vi "多参10分钟延时启动.vi"(11 "启动采配水？":bool) -> ()   [LabVIEW 2016]
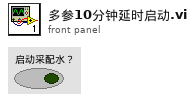
[diagram p1: front panel]
types:
  T1 = cluster{"命令":string, cluster{"starting address":u16, "holding register value":u16}}
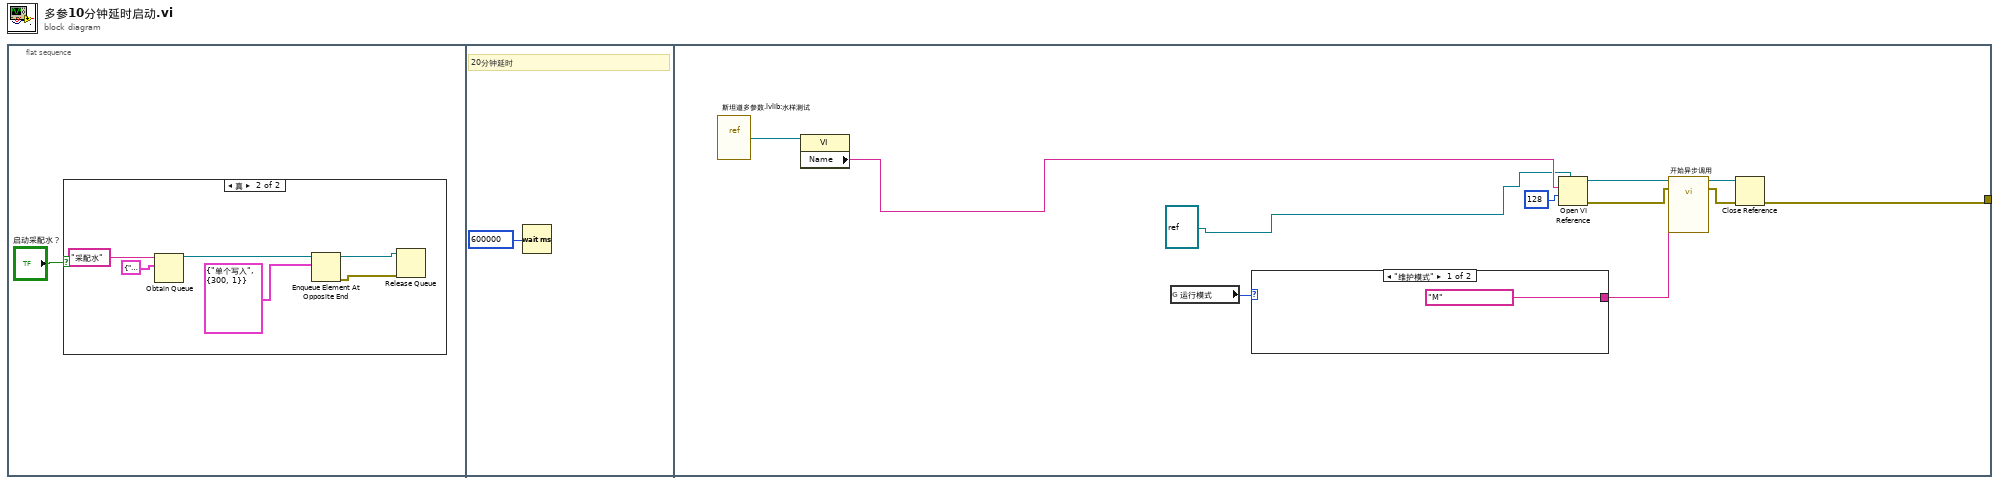
[diagram p0: block diagram]
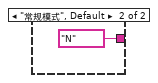
[diagram p3: hidden frame]
diagram:
  n1 = flat-sequence {
    tunnel: [w10] -> _
    frame #0 {
      n2 = case shown="真" "启动采配水？" {
        frame False {
        }
        frame True {
          n3 = Obtain Queue(name (unnamed)="采配水" ("名称（未命名）"), element data type=cluster{"命令":string, "数据":variant} {"命令"="", "数据"=variant}) -> (queue out=w4:refnum<queue>)  [unwired: 3 in, 2 out]
          n4 = Enqueue Element At Opposite End(queue=w4, element=T1 {"命令"="单个写入", {"starting address"=300, "holding register value"=1}} ("元素")) -> (queue out=w3:refnum<queue>, error out=w2:errorcluster)  [unwired: 2 in, 1 out]
          n5 = Release Queue(queue=w3, error in (no error)=w2) -> ()  [unwired: 1 in, 3 out]
        }
      }
    }
    frame #1 {
      # "20分钟延时"
      n6 = Wait (ms)(milliseconds to wait=u32 600000 ("等待时间（毫秒）")) -> ()  [unwired: 1 out]
    }
    frame #2 {
      n7 = vi-ref "斯坦道多参数.lvlib:水样测试.vi"() -> (w19:refnum<vi>)
      n8 = property class="VI"(reference=w19) -> ("Name"=w18:string)  [unwired: 1 in, 2 out]
      n9 = global read "系统设置全局变量.vi" "运行模式"() -> (w14:enum16{"维护模式", "常规模式", "应急模式", "质控模式"})
      n10 = case shown="\"维护模式\"" w14 {
        tunnel: ["M" ("数据标记表") "N" ("数据标记表")] -> w13
        frame "维护模式" {
        }
        frame "常规模式", Default {
        }
      }
      n11 = Open VI Reference(type specifier VI Refnum (for type only)=refnum<vi> refnum, vi path=w18, options=128 ("选项")) -> (vi reference=w16:refnum<vi>, error out=w9:errorcluster)  [unwired: 3 in]
      n12 = call-by-ref "开始异步调用"(reference=w16, error in=w9, "数据标记表"=w13) -> (reference out=w15:refnum<vi>, error out=w11:errorcluster)  [unwired: 11 in]
      n13 = Close Reference(reference=w15, error in (no error)=w11) -> (error out=w10:errorcluster)
    }
  }
